vi "FindClassInProject.vi"(8 "error in (no error)":errorcluster, 10 "Name":string) -> (0 "error out":errorcluster, 1 "Found":bool, 2 "LVClassLibrary Refnum":refnum<vi>)   [LabVIEW 2013, in "GenLVOOP.lvclass"]
uses:
  GenLVOOP.lvclass
  ProjectHandler/RefNums.vi
  ProjectHandler.lvlib
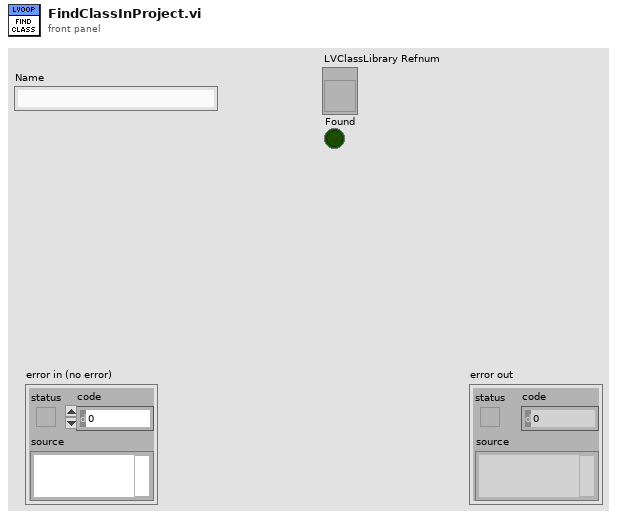
[diagram p1: front panel]
types:
  T1 = cluster{"App":refnum<vi>, "Project":refnum<vi>, "My Computer":refnum<vi>}
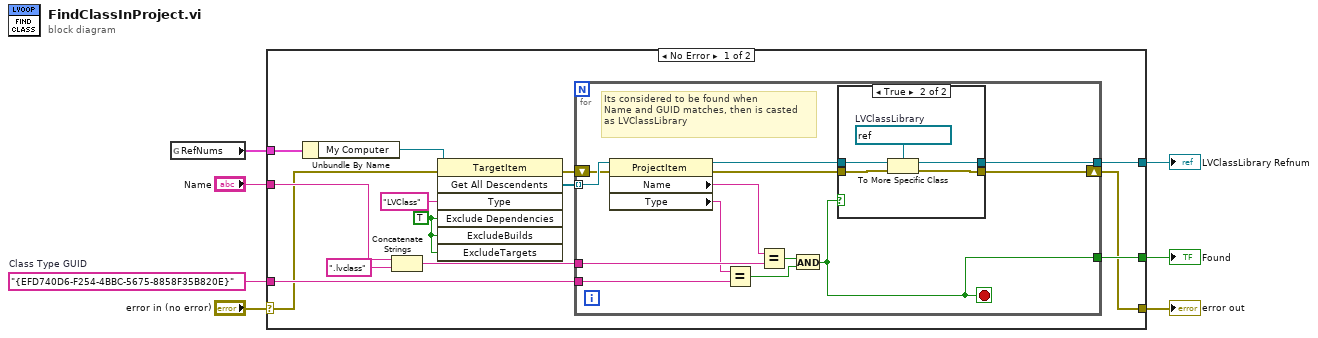
[diagram p0: block diagram]
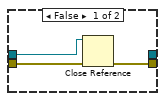
[diagram p2: hidden frame]
diagram:
  w4 = "{EFD740D6-F254-4BBC-5675-8858F35B820E}"  # Class Type GUID
  n1 = global read "RefNums.vi" "RefNums"() -> (w5:T1)
  n2 = case shown="No Error" "error in (no error)" {
    selector: "error in (no error)" -> [w10 w43]
    tunnel: [w14 w43] -> w6
    tunnel: w5 -> [w21 _]
    tunnel: w4 -> [w20 _]
    tunnel: [w19 _] -> w3
    tunnel: [w18 _] -> w2
    tunnel: "Name" -> [w15 _]
    frame No Error {
      w9 = TRUE ("ExcludeDependencies")
      n3 = Unbundle By Name(w21) -> ("My Computer"=w13:refnum<vi>)
      n4 = Concatenate Strings(w15, ".lvclass" ("string")) -> (w17:string)
      n5 = invoke class="TargetItem" method="Get All Descendents"(reference=w13, error in=w10, "Type"="LVClass", "Exclude Dependencies"=w9, "ExcludeBuilds"=w9, "ExcludeTargets"=w9) -> (error out=w11:errorcluster, "All Descendents"=w12:refnum<vi>[])  [unwired: 1 in, 5 out]
      n6 = for {
        tunnel: w12 -> [w33] mode=indexing
        tunnel: w20 -> [w34]
        tunnel: w17 -> [w32]
        tunnel: [w29] -> w19
        tunnel: [w28] -> w18
        shift-right: [w22] -> w14
        shift-left: w11 -> [w27]
        stop <- w28 stop-if-true
        # "Its considered to be found when \nName and GUID matches, then is casted\nas LVClassLibrary"
        n7 = property class="ProjectItem"(reference=w33, error in=w27) -> (reference out=w24:refnum<vi>, error out=w23:errorcluster, "Name"=w26:string, "Type"=w25:string)
        n8 = Equal?(x=w25, y=w34) -> (x = y?=w30:bool)
        n9 = Equal?(x=w26, y=w32) -> (x = y?=w31:bool)
        n10 = And(x=w31, y=w30) -> (x .and. y?=w28:bool)
        n11 = case shown="True" w28 {
          tunnel: w24 -> [w37 w41]
          tunnel: [_ w40] -> w29
          tunnel: w23 -> [w36 w39]
          tunnel: [w35 w38] -> w22
          frame False {
            n12 = Close Reference(reference=w37, error in (no error)=w36) -> (error out=w35:errorcluster)
          }
          frame True {
            w42 = refnum<vi> refnum  # LVClassLibrary
            n13 = To More Specific Class(target class=w42, reference=w41, error in=w39) -> (specific class reference=w40:refnum<vi>, error out=w38:errorcluster)
          }
        }
      }
    }
    frame Error {
    }
  }
  "error out" <- w6
  "LVClassLibrary Refnum" <- w3
  "Found" <- w2
